vi "Manual Triggered B-Scan.vi"() -> ()   [LabVIEW 2012]
uses:
  LabVIEW/user.lib/SpectralRadar.llb/Processing Flag Selection.ctl
  LabVIEW/user.lib/SpectralRadar.llb/set Scan Output.vi
  LabVIEW/user.lib/SpectralRadar.llb/display Data 2D.vi
  LabVIEW/user.lib/SpectralRadar.llb/OCT Device.lvclass
  LabVIEW/user.lib/SpectralRadar.llb/Processing.lvclass
  LabVIEW/user.lib/SpectralRadar.llb/Probe.lvclass
  LabVIEW/user.lib/SpectralRadar.llb/Scan Pattern.lvclass
  LabVIEW/user.lib/SpectralRadar.llb/Raw Data.lvclass
  LabVIEW/user.lib/SpectralRadar.llb/Data.lvclass
panel:
  out "B-scan display":dbl[][](graph)
  in  "A-scans / B-scan":i32=512
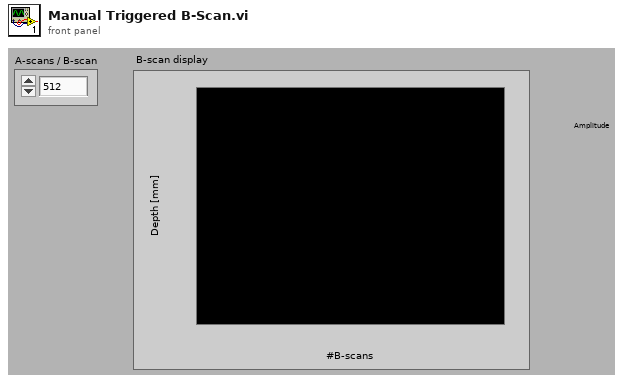
[diagram p1: front panel]
types:
  T1 = typedef "Processing.lvclass/Processing Flag Selection.ctl" = enum16{"Use Offset Errors", "Remove DC Spectrum", "Remove Advanced DC Spectrum", "Use Apodization", "Use Scan For Apodization", "Filter Undersampled Signals", "Use Dispersion Compensation", "Use Dechirp", "Use Extended Adjust", "Full Range Output", "Filter DC", "Autocorrelation Compensation", "DEFR", "Only Windowing", "Remove Fixed Pattern"}
  T2 = enum16{"Asynchronous Continuous", "Asynchronous Finite", "Synchronous"}
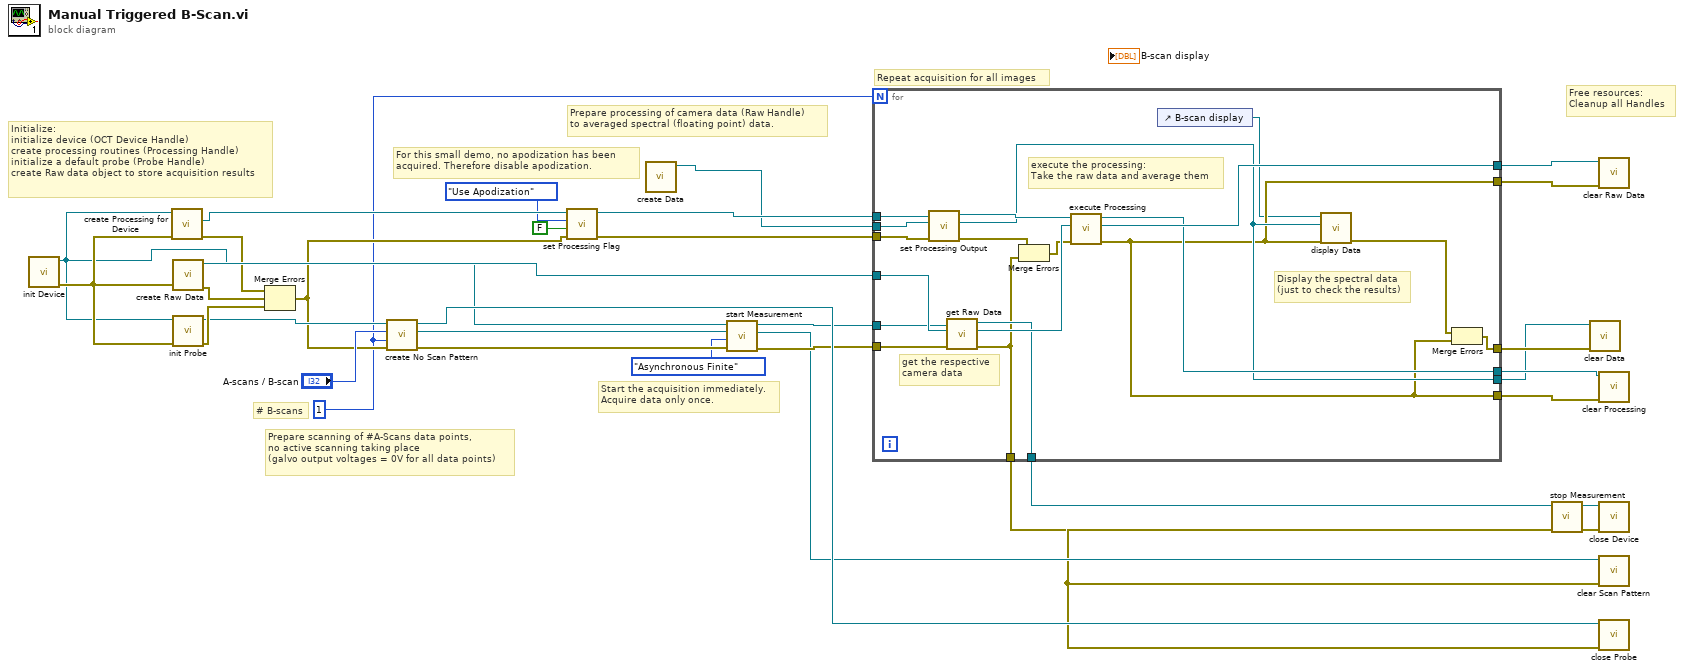
[diagram p0: block diagram]
diagram:
  w5 = 1 ("Number of Scand")
  # "Repeat acquisition for all images"
  # "For this small demo, no apodization has been \nacquired. Therefore disable apodization."
  # "# B-scans"
  # "Free resources:\nCleanup all Handles"
  # "Prepare processing of camera data (Raw Handle)\nto averaged spectral (floating point) data."
  # "Start the acquisition immediately.\nAcquire data only once."
  # "Prepare scanning of #A-Scans data points,\nno active scanning taking place \n(galvo output voltages = 0V for all data points)"
  # "Initialize:\ninitialize device (OCT Device Handle)\ncreate processing routines (Processing Handle)\ninitialize a default probe (Probe Handle)\ncreate Raw data object to store acquisition results"
  n1 = call "init Device.vi"() -> ("error out"=w33:errorcluster, "OCTDevice"=w4:refnum<class "OCT Device.lvclass">)  [unwired: 6 in]
  n2 = call "create Processing for Device.vi"("error in (no error)"=w33, "OCTDevice"=w4) -> ("error out"=w31:errorcluster, "Processing"=w12:refnum<class "Processing.lvclass">)  [unwired: 3 in, 1 out]
  n3 = call "create Raw Data.vi"("error in (no error)"=w33) -> ("error out"=w30:errorcluster, "Raw Data"=w32:refnum<class "Raw Data.lvclass">)  [unwired: 5 in]
  n4 = call "init Probe.vi"("error in (no error)"=w33, "OCT Device"=w4) -> ("error out"=w26:errorcluster, "GalvoControl"=w16:refnum<class "Probe.lvclass">)  [unwired: 4 in]
  n5 = Merge Errors(w31, w30, w26) -> (w8:errorcluster)
  n6 = call "create No Scan Pattern.vi"("error in (no error)"=w8, "Number of Scans"=w5, "AScans"="A-scans / B-scan", "Probe"=w16) -> ("error out"=w29:errorcluster, "Scan Pattern"=w28:refnum<class "Scan Pattern.lvclass">, "Probe"=w27:refnum<class "Probe.lvclass">)  [unwired: 1 in]
  n7 = call "set Processing Flag.vi"("error in (no error)"=w8, "Flag"=FALSE, "Processing Flag Selection"=Processing_Flag_Selection."Use Apodization", "Processing"=w12) -> ("error out"=w7:errorcluster, "Processing"=w11:refnum<class "Processing.lvclass">)  [unwired: 2 in]
  n8 = call "create Data.vi"() -> ("Data"=w3:refnum<class "Data.lvclass">)  [unwired: 6 in, 1 out]
  n9 = call "start Measurement.vi"("error in (no error)"=w29, "Acquisition Type"=T2."Asynchronous Finite", "Scan Pattern"=w28, "OCTDevice"=w4) -> ("error out"=w23:errorcluster, "Scan Pattern"=w20:refnum<class "Scan Pattern.lvclass">, "OCTDevice"=w24:refnum<class "OCT Device.lvclass">)  [unwired: 1 in]
  n10 = for {
    N: w5 -> [_]
    tunnel: w32 -> [w52]
    tunnel: w3 -> [w51]
    tunnel: w24 -> [w50]
    tunnel: w23 -> [w49]
    tunnel: [w46] -> w22
    tunnel: [w44] -> w2
    tunnel: [w43] -> w21
    tunnel: [w41] -> w17
    tunnel: [w39] -> w14
    tunnel: [w38] -> w1
    tunnel: [w35] -> w13
    tunnel: w11 -> [w37]
    tunnel: w7 -> [w36]
    tunnel: [w35] -> w6
    # "Display the spectral data\n(just to check the results)"
    # "execute the processing:\nTake the raw data and average them"
    # "get the respective \ncamera data"
    n11 = call-poly "set Processing Output.vi"("error in (no error)"=w36, "Data"=w51, "Processing"=w37) -> ("error out"=w42:errorcluster, "Data"=w38:refnum<class "Data.lvclass">, "Processing"=w48:refnum<class "Processing.lvclass">)  [unwired: 2 in]
    n12 = call "get Raw Data.vi"("error in (no error)"=w49, "RawData in"=w52, "OCTDevice in"=w50) -> ("error out"=w41:errorcluster, "RawData out"=w47:refnum<class "Raw Data.lvclass">, "OCTDevice out"=w43:refnum<class "OCT Device.lvclass">)  [unwired: 2 in]
    n13 = Merge Errors(w42, w41) -> (w40:errorcluster)
    n14 = call "execute Processing.vi"("error in (no error)"=w40, "Raw Data"=w47, "Processing"=w48) -> ("error out"=w35:errorcluster, "Raw Data"=w46:refnum<class "Raw Data.lvclass">, "Processing"=w39:refnum<class "Processing.lvclass">)  [unwired: 2 in]
    n15 = control-ref of="B-scan display"() -> (w34:refnum<vi>)
    n16 = call-poly "display Data.vi"("error in (no error)"=w35, "Data in"=w38, "IntGraph Refnum"=w34) -> ("error out"=w45:errorcluster)  [unwired: 2 in, 2 out]
    n17 = Merge Errors(w45, w35) -> (w44:errorcluster)
  }
  n18 = call "stop Measurement.vi"("error in (no error)"=w17, "OCTDevice"=w21) -> ("error out"=w18:errorcluster, "OCTDevice"=w19:refnum<class "OCT Device.lvclass">)  [unwired: 4 in]
  n19 = call "clear Data.vi"("error in (no error)"=w2, "Data"=w1) -> ()  [unwired: 5 in, 1 out]
  n20 = call "clear Raw Data.vi"("error in (no error)"=w13, "Raw Data"=w22) -> ()  [unwired: 5 in, 1 out]
  n21 = call "clear Processing.vi"("error in (no error)"=w6, "Processing"=w14) -> ()  [unwired: 5 in, 1 out]
  n22 = call "close Device.vi"("error in (no error)"=w18, "OCTDevice"=w19) -> ()  [unwired: 5 in, 1 out]
  n23 = call "clear Scan Pattern.vi"("error in (no error)"=w18, "Scan Pattern in"=w20) -> ()  [unwired: 5 in, 1 out]
  n24 = call "close Probe.vi"("error in (no error)"=w18, "GalvoControl"=w27) -> ()  [unwired: 5 in, 1 out]
